vi "Fetch Waveforms.vi"(8 "error in (no error)":errorcluster, 11 "Scope Base in":refnum<class "Scope Base.lvclass">) -> (0 "error out":errorcluster, 3 "Scope Base out":refnum<class "Scope Base.lvclass">)   [LabVIEW 2023, in "Scope.lvlib" / "Scope Base.lvlib" / "Scope Base.lvclass"]
uses:
  Scope Base.lvclass
  Interfaces/IConfigure Scope/IConfigure Scope.lvclass
  Scope Base.lvclass/Scope Base.ctl
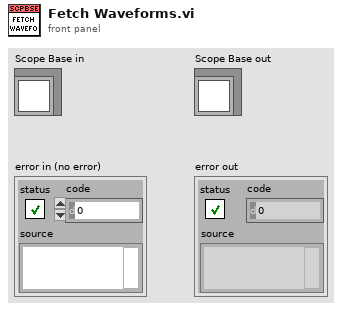
[diagram p1: front panel]
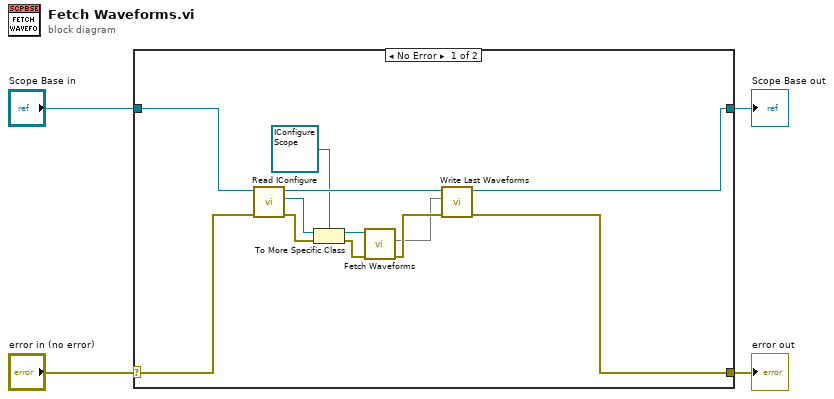
[diagram p0: block diagram]
diagram:
  n1 = case shown="No Error" "error in (no error)" {
    selector: "error in (no error)" -> [w16 w18]
    tunnel: [w12 w18] -> w3
    tunnel: [w10 w17] -> w1
    tunnel: "Scope Base in" -> [w15 w17]
    frame No Error {
      n2 = call "Read IConfigure.vi"("error in (no error)"=w16, "Scope Base in"=w15) -> ("error out"=w8:errorcluster, "IConfigureScope"=w14:refnum<class "IConfigure.lvclass">, "Scope Base out"=w11:refnum<class "Scope Base.lvclass">)  [unwired: 7 in]
      n3 = To More Specific Class(target class=refnum<class "IConfigure Scope.lvclass"> refnum ("IConfigure Scope.lvclass"), reference=w14, error in=w8) -> (specific class reference=w6:refnum<class "IConfigure Scope.lvclass">, error out=w7:errorcluster)
      n4 = call-dynamic "Fetch Waveforms.vi"("error in"=w7, "IConfigure Scope in"=w6) -> ("error out"=w13:errorcluster, "Last Waveforms"=w9:map{u8, waveform(dbl)})  [unwired: 7 in, 1 out]
      n5 = call "Write Last Waveforms.vi"("error in (no error)"=w13, "Last Waveforms"=w9, "Scope Base in"=w11) -> ("error out"=w12:errorcluster, "Scope Base out"=w10:refnum<class "Scope Base.lvclass">)  [unwired: 7 in]
    }
    frame Error {
    }
  }
  "error out" <- w3
  "Scope Base out" <- w1
